vi "GetUIRef.vi"(8 "error in (no error)":errorcluster, 11 "View in":refnum<class "View.lvclass">) -> (0 "error out":errorcluster, 2 "UIRef":refnum<vi>, 3 "View out":refnum<class "View.lvclass">)   [LabVIEW 2020, in "Page2.lvlib" / "View.lvclass"]
uses:
  View.lvclass
  UI.vi
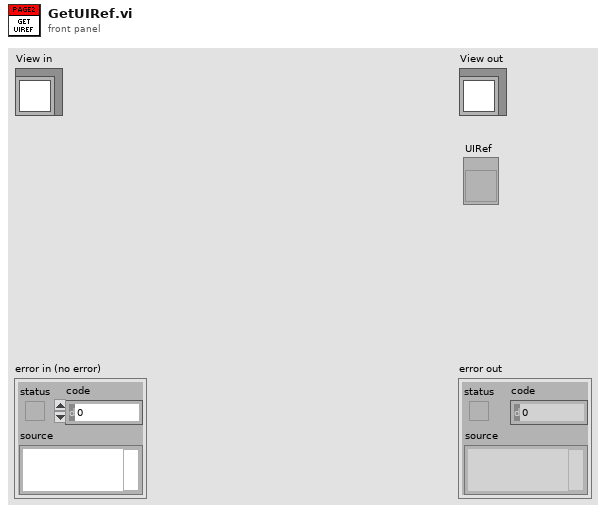
[diagram p1: front panel]
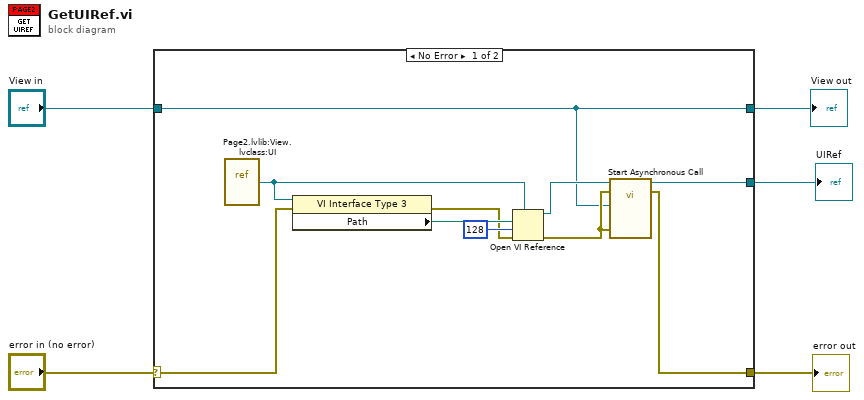
[diagram p0: block diagram]
diagram:
  n1 = case shown="No Error" "error in (no error)" {
    selector: "error in (no error)" -> [w9 w17]
    tunnel: [w15 w17] -> w2
    tunnel: [w7 w16] -> w4
    tunnel: "View in" -> [w7 w16]
    tunnel: [w6 _] -> w1
    frame No Error {
      n2 = vi-ref "Page2.lvlib:View.lvclass:UI.vi"() -> (w11:refnum<vi>)
      n3 = property class="VI Interface Type 3"(reference=w11, error in=w9) -> (error out=w10:errorcluster, "Path"=w14:path)  [unwired: 1 out]
      n4 = Open VI Reference(type specifier VI Refnum (for type only)=w11, vi path=w14, options=128, error in (no error)=w10) -> (vi reference=w12:refnum<vi>, error out=w8:errorcluster)  [unwired: 2 in]
      n5 = call-by-ref "Start Asynchronous Call"(reference=w12, error in=w8, 8:"error in (no error)"=w8, "View in"=w7) -> (reference out=w6:refnum<vi>, error out=w15:errorcluster)  [unwired: 8 in, 2 out]
    }
    frame Error {
    }
  }
  "error out" <- w2
  "View out" <- w4
  "UIRef" <- w1
